vi "test_ThreeSessThreePinTwoInstrTwoSiteReservation_CallGetConnectionsFromPinForAllDcPowerPinsAllSites_ReturnsThreeConnections.vi"(8 "error in":errorcluster) -> (0 "error out":errorcluster, 2 "result":string, 3 "pass":bool)   [LabVIEW 2020, in "MeasurementServerTests.lvlib"]
uses:
  MeasurementServerTests.lvlib
  Runtime/MeasurementLink Session Management/Session Reservation/Connection.ctl
  Runtime/MeasurementLink Session Management/Session Reservation/Session Reservation.lvclass
  Runtime/MeasurementLink Session Management/Session Reservation/Connection with Session.ctl
  b3e5c3be-b7a7-4b6e-86ee-709eea9cb752.vi
  514a39f3-05c6-4c8c-919b-303d9a210aef.vi
  481e2142-dde9-4265-ba9c-fc6a4d123327.vi
  da43ad04-91ae-4dbc-8eb3-60d6b08c7e97.vi
  e462a96d-9dce-4a61-b4bd-fba70dd973b3.vi
  Runtime/MeasurementLink niDCPower/Instrument/Instrument.lvclass
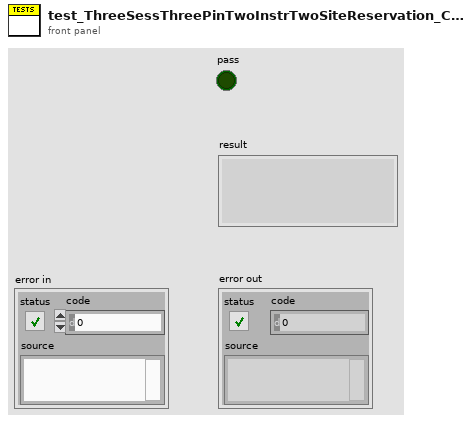
[diagram p1: front panel]
types:
  T1 = typedef "MeasurementLink Session Management.lvlib/Session Reservation.lvclass/Connection.ctl" = cluster{"pin or relay name":string, "site":i32, "instrument type id":string, "channel":string}
  T2 = typedef "MeasurementLink Session Management.lvlib/Session Reservation.lvclass/Connection with Session.ctl" = cluster{"connection":T1, "session":variant}
  T3 = typedef "MeasurementLink Session Management.lvlib/Session Reservation.lvclass/Data.ctl" = cluster{"session and driver infos":T4[], "pin or relay names":string[]}
  T4 = typedef "MeasurementLink Session Management.lvlib/Session Reservation.lvclass/Session and Driver Info.ctl" = cluster{"session info":T5, "session":variant}
  T5 = typedef "MeasurementLink Session Management Client.lvlib/ni_measurementlink_sessionmanagement_v1_SessionInformation.ctl" = cluster{"session":T6, "resource_name":string, "channel_list":string, "instrument_type_id":string, "session_exists":bool, "channel_mappings":T7[]}
  T6 = typedef "MeasurementLink Session Management Client.lvlib/nidevice_grpc_Session.ctl" = cluster{"name":string}
  T7 = typedef "MeasurementLink Session Management Client.lvlib/ni_measurementlink_sessionmanagement_v1_ChannelMapping.ctl" = cluster{"pin_or_relay_name":string, "site":i32, "channel":string}
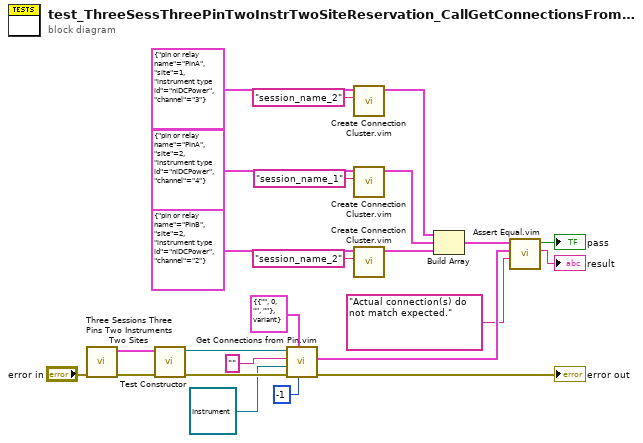
[diagram p0: block diagram]
diagram:
  n1 = call "Three Sessions Three Pins Two Instruments Two Sites.vi"("error in"="error in") -> ("error out"=w19:errorcluster, "data out"=w18:T3)  [unwired: 9 in]
  n2 = call "Test Constructor.vi"("error in"=w19, "data"=w18) -> ("error out"=w9:errorcluster, "Session Reservation out"=w11:refnum<class "Session Reservation.lvclass">)  [unwired: 8 in]
  n3 = call "Get Connections from Pin.vim"("site"=-1, "connection type"=T2 {"connection"={"pin or relay name"="", "site"=0, "instrument type id"="", "channel"=""}, "session"=variant} ("connection"), "error in"=w9, "instrument"=refnum<class "Instrument.lvclass"> refnum ("MeasurementLink niDCPower.lvlib:Instrument.lvclass"), "pin or relay name"="", "session reservation in"=w11) -> ("error out"=→"error out":errorcluster, "connections"=w23:T2[])  [unwired: 3 in, 1 out]
  n4 = call "Create Connection Cluster.vim"("session in"="session_name_2", "hardware independent connection in"=T1 {"pin or relay name"="PinA", "site"=1, "instrument type id"="niDCPower", "channel"="3"} ("connection")) -> ("connection out"=w17:T2)  [unwired: 9 in]
  n5 = call "Create Connection Cluster.vim"("session in"="session_name_1", "hardware independent connection in"=T1 {"pin or relay name"="PinA", "site"=2, "instrument type id"="niDCPower", "channel"="4"} ("connection")) -> ("connection out"=w6:T2)  [unwired: 9 in]
  n6 = call "Create Connection Cluster.vim"("session in"="session_name_2", "hardware independent connection in"=T1 {"pin or relay name"="PinB", "site"=2, "instrument type id"="niDCPower", "channel"="2"} ("connection")) -> ("connection out"=w2:T2)  [unwired: 9 in]
  n7 = Build Array(w17, w6, w2) -> (w16:T2[])
  n8 = call "Assert Equal.vim"("failure message"="Actual connection(s) do not match expected.", "actual value"=w23, "expected value"=w16) -> ("message"=→"result":string, "equal?"=→"pass":bool)  [unwired: 7 in]
